vi "Close.vi"(8 "error in (no error)":errorcluster {"code" format="%x"}, 11 "deviceId":i32) -> (0 "error out":errorcluster {"code" format="%x"})   [LabVIEW 2020, in "Keyence CL-3000.lvlib"]
doc: "Performs an instrument error query before terminating the software connection to the instrument."
uses:
  Keyence CL-3000.lvlib
  Private/enums/Function Name.ctl
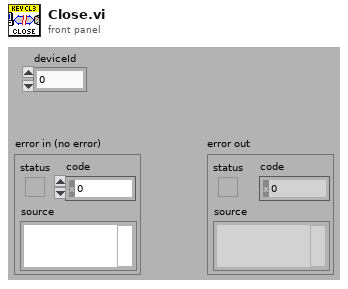
[diagram p1: front panel]
types:
  T1 = typedef "Keyence CL-3000.lvlib/Function Name.ctl" = enum16{"Initialize", "Close", "CL3IF_GetMeasurementData", "CL3IF_GetTrendIndex", "CL3IF_GetTrendData", "CL3IF_GetStorageIndex", "CL3IF_GetStorageData", "CL3IF_AutoZeroMulti", "CL3IF_AutoZeroGroup", "CL3IF_TimingMulti", "CL3IF_TimingGroup", "CL3IF_ResetMulti", "CL3IF_ResetGroup", "CL3IF_LightControl", "CL3IF_MeasurementControl", "CL3IF_SwitchProgram", "CL3IF_GetProgramNo", "CL3IF_StartStorage", "CL3IF_StopStorage", "CL3IF_ClearStorageData", "CL3IF_GetPulseCount", "CL3IF_ResetPulseCount", "CL3IF_GetLightWaveform"}
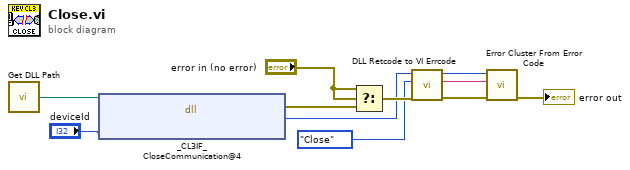
[diagram p0: block diagram]
diagram:
  n1 = call "Get DLL Path.vi"() -> ("DLL Path"=w5:path)  [unwired: 1 in]
  n2 = dll-call lib="C:/Program Files (x86)/National Instruments/LabVIEW 2018/instr.lib/Keyence CL-3000/CL3_IF.dll" fn="_CL3IF_CloseCommunication@4"(path in=w5, "deviceId"="deviceId") -> (error out=w3:errorcluster, "RC"=w4:i32)  [unwired: 3 in, 1 out]
  n3 = Select(t="error in (no error)", s="error in (no error)", f=w3) -> (s? t:f=w10:errorcluster)
  n4 = call "DLL Retcode to VI Errcode.vi"("error in (no error)"=w10, "Function Name"=Function_Name."Close", "DLL Retcode"=w4) -> ("error out"=w8:errorcluster, "ErrorMessage"=w2:string, "VI Errcode"=w9:i32)  [unwired: 6 in]
  n5 = call <vilib>:"Error Cluster From Error Code.vi"("error in (no error)"=w8, "error message (\"\")"=w2, "error code (0)"=w9) -> ("error out"=→"error out":errorcluster)  [unwired: 6 in]
